vi "Display Preview (SubVI).vi"(0 "Display Data":T3, 5 "Image Size":T1={"Height"=512, "Width"=512} {"Width" step=8; "Height" step=8}) -> (14 "Image Out":T2)   [LabVIEW 2020]
uses:
  Controls (HOST)/Image Size.ctl
  Controls (HOST)/Data to Disk Bundle.ctl
  <vilib>/vision/Image Controls.llb/IMAQ Image.ctl
  <vilib>/vision/NI_Vision_Development_Module.lvlib
panel:
  in  "Image Size 2":T1={"Height"=512, "Width"=512} {"Width" step=8; "Height" step=8}
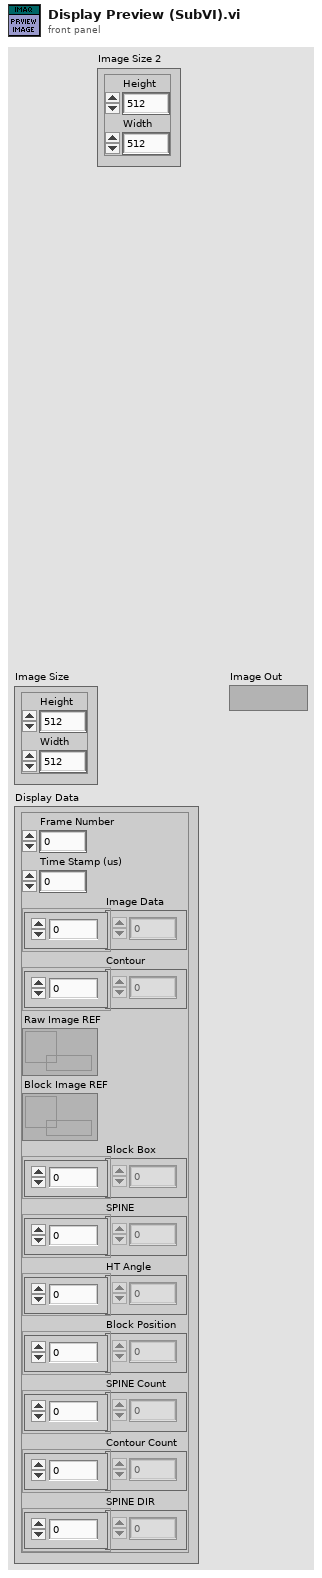
[diagram p1: front panel]
types:
  T1 = typedef "Image Size.ctl" = cluster{"Height":u16, "Width":u16}
  T2 = typedef "IMAQ Image.ctl" = refnum<image>
  T3 = typedef "Data to Disk Bundle.ctl" = cluster{"Frame Number":u64, "Time Stamp (us)":u64, "Image Data":u64[], "Contour":u32[], "Raw Image REF":refnum<data-value>, "Block Image REF":refnum<data-value>, "Block Box":u64[], "SPINE":u32[], "HT Angle":u64[], "Block Position":u64[], "SPINE Count":u32[], "Contour Count":u32[], "SPINE DIR":u8[]}
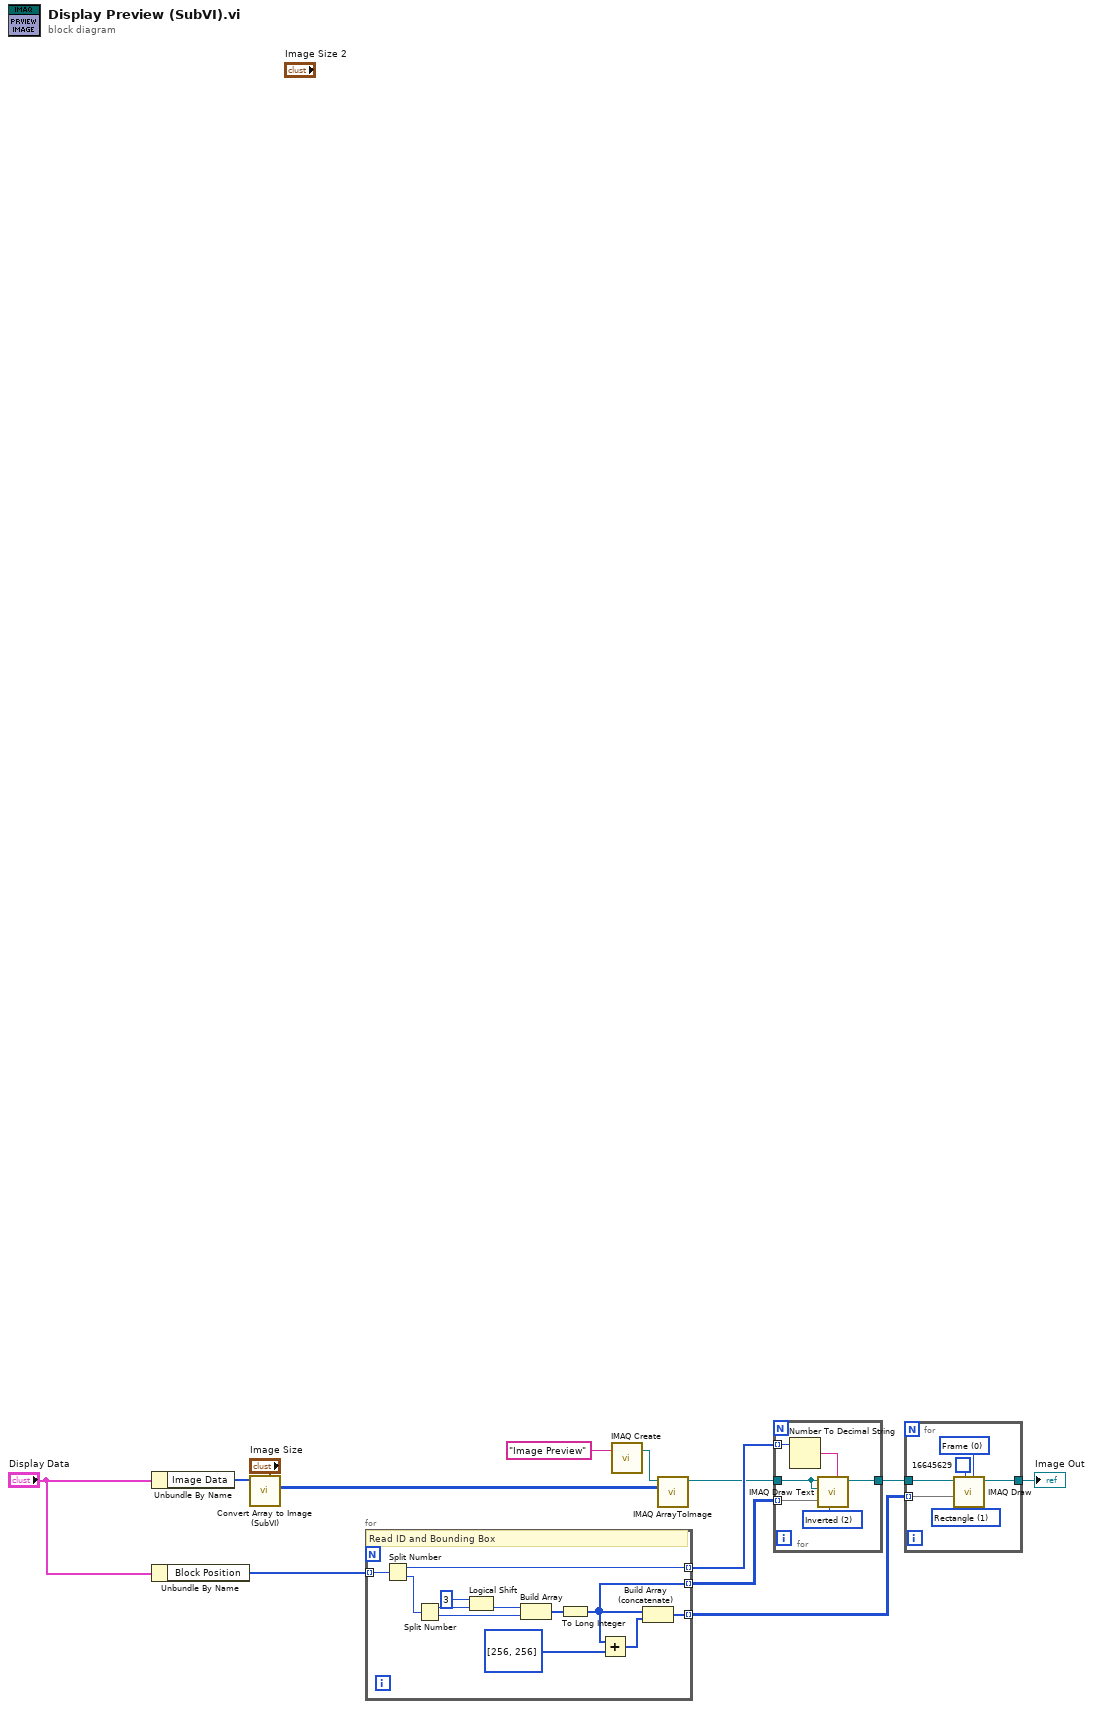
[diagram p0: block diagram]
diagram:
  n1 = Unbundle By Name("Display Data") -> ("Image Data"=w11:u64[])
  n2 = Unbundle By Name("Display Data") -> ("Block Position"=w8:u64[])
  n3 = call "Convert Array to Image (SubVI).vi"("Image Size"="Image Size", "Image Array In"=w11) -> ("Image Array Out"=w9:u8[][])  [unwired: 9 in]
  n4 = for {
    tunnel: w8 -> [w25] mode=indexing
    tunnel: [w24] -> w5 mode=indexing
    tunnel: [w17] -> w7 mode=indexing
    tunnel: [w16] -> w6 mode=indexing
    # "Read ID and Bounding Box"
    n5 = Split Number(x=w25) -> (hi(x)=w24:u32, lo(x)=w23:u32)
    n6 = Split Number(x=w23) -> (hi(x)=w22:u16, lo(x)=w21:u16)
    n7 = Logical Shift(y=i16 3, x=w22) -> (x << y=w15:u16)
    n8 = Build Array(w15, w21) -> (w18:u16[])
    n9 = To Long Integer(number=w18) -> (32bit integer=w16:i32[])
    n10 = Add(x=w16, y=i32[] [256, 256]) -> (x+y=w19:i32[])
    n11 = Build Array (concatenate)(w16, w19) -> (w17:i32[])
  }
  n12 = call "IMAQ Create"("Image Name"="Image Preview") -> ("New Image"=w10:T2)  [unwired: 4 in, 1 out]
  n13 = call "IMAQ ArrayToImage"("Image Pixels (U8)"=w9, "Image"=w10) -> ("Image Out"=w4:T2)  [unwired: 8 in, 1 out]
  n14 = for {
    tunnel: w6 -> [w29] mode=indexing
    tunnel: w5 -> [w27] mode=indexing
    tunnel: w4 -> [w31]
    tunnel: [w30] -> w3
    w28 = 2 items=["White", "Black", "Inverted", "Black on White", "White on Black"] ("Color")
    n15 = Number To Decimal String(number=w27) -> (decimal integer string=w26:string)  [unwired: 1 in]
    n16 = call "IMAQ Draw Text"("String"=w26, "Insertion Point"=w29, "Color"=w28, "Image Dst"=w31, "Image Src"=w31) -> ("Image Dst Out"=w30:T2)  [unwired: 3 in, 3 out]
  }
  n17 = for {
    tunnel: w7 -> [w35] mode=indexing
    tunnel: w3 -> [w37]
    tunnel: [w36] -> w2
    w33 = u16 0 items=["Frame", "Paint", "Invert Frame", "Invert Paint"] ("Draw Mode")
    w34 = u16 1 items=["Line", "Rectangle", "Oval"] ("Shape to draw")
    n18 = call "IMAQ Draw"("Draw Mode"=w33, "Shape to draw"=w34, "Pixel Color"=u32 16645629, "Coordinates"=w35, "Image Dst"=w37, "Image Src"=w37) -> ("Image Dst Out"=w36:T2)  [unwired: 4 in, 1 out]
  }
  "Image Out" <- w2
